vi "ROI parser.vi"(4 "# pixels in an ablation spot":i32, 5 "ROI Height in pixel":dbl, 6 "Heigth step size in pixel":dbl, 7 "ROI (8 bit image)":u8[][](array[numeric]), 8 "Ablation spot width":dbl, 9 "ROI Width in pixel":dbl, 10 "Sampling\nPrecision":dbl, 11 "Ablation spot heigth":dbl) -> (3 "Parsed array":bool[][](array[boolean]))   [LabVIEW 2016]
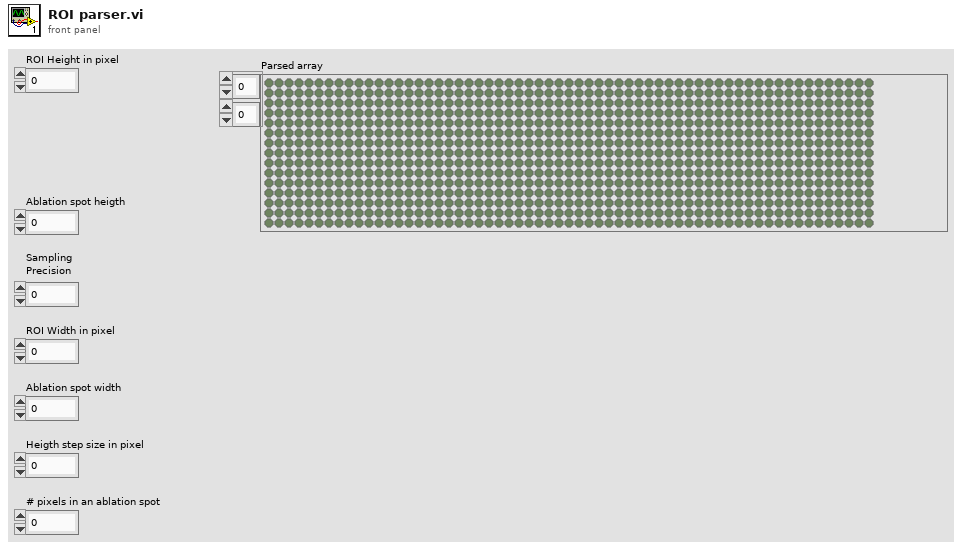
[diagram p1: front panel]
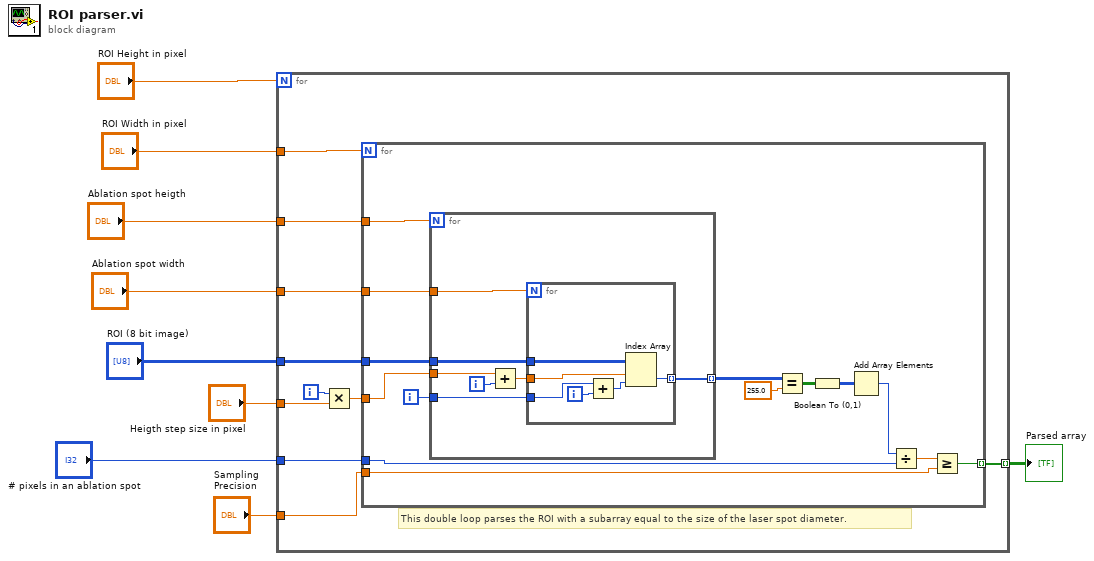
[diagram p0: block diagram]
diagram:
  n1 = for {
    N: "ROI Height in pixel" -> [_]
    tunnel: "ROI (8 bit image)" -> [w19]
    tunnel: "ROI Width in pixel" -> [w18]
    tunnel: "Ablation spot heigth" -> [w17]
    tunnel: [w16] -> w1 mode=indexing
    tunnel: "Heigth step size in pixel" -> [w13]
    tunnel: "Ablation spot width" -> [w12]
    tunnel: "# pixels in an ablation spot" -> [w11]
    tunnel: "Sampling\nPrecision" -> [w10]
    i -> [w15]
    # "This double loop parses the ROI with a subarray equal to the size of the laser spot diameter."
    n2 = Multiply(x=w15, y=w13) -> (x*y=w14:dbl)
    n3 = for {
      N: w18 -> [_]
      tunnel: w17 -> [w28]
      tunnel: w14 -> [w30]
      tunnel: w19 -> [w29]
      tunnel: [w27] -> w16 mode=indexing
      tunnel: w12 -> [w23]
      tunnel: w11 -> [w22]
      tunnel: w10 -> [w21]
      i -> [w25]
      n4 = for {
        N: w28 -> [_]
        tunnel: w29 -> [w40]
        tunnel: [w39] -> w24 mode=indexing
        tunnel: w23 -> [w38]
        tunnel: w30 -> [w37]
        tunnel: w25 -> [w34]
        i -> [w36]
        n5 = Add(x=w37, y=w36) -> (x+y=w35:dbl)
        n6 = for {
          N: w38 -> [_]
          tunnel: w40 -> [w46]
          tunnel: [w45] -> w39 mode=indexing
          tunnel: w35 -> [w44]
          tunnel: w34 -> [w42]
          i -> [w43]
          n7 = Add(x=w42, y=w43) -> (x+y=w41:i32)
          n8 = Index Array(array=w46, index (row)=w44, index (col)=w41) -> (element=w45:u8)
        }
      }
      n9 = Equal?(x=w24, y=255.0) -> (x = y?=w32:bool[][])
      n10 = Boolean To (0,1)(Boolean=w32) -> (0, 1=w31:i16[][])
      n11 = Add Array Elements(numeric array=w31) -> (sum=w20:i16)
      n12 = Divide(x=w20, y=w22) -> (x/y=w26:dbl)
      n13 = Greater Or Equal?(x=w26, y=w21) -> (x >= y?=w27:bool)
    }
  }
  "Parsed array" <- w1
